vi "Handle Menu Selection.vi"(6 "Coords":T1, 8 "error in (no error)":errorcluster, 9 "Item Tag":string, 10 "Tree Refnum":refnum<vi>, 11 "Process Builder View in":refnum<class "Process Builder View.lvclass">) -> (0 "error out":errorcluster, 3 "Process Builder View out":refnum<class "Process Builder View.lvclass">)   [LabVIEW 2019, in "Process Builder View.lvclass"]
uses:
  <vilib>/gpm_packages/@cs/Car-wash/Source/Process Builder View/Process Builder View.lvclass
  C:/Program Files/National Instruments/LabVIEW 2019/vi.lib/gpm_packages/@cs/Test-executive-builder/Source/Test Executive Builder View/Test Executive Builder View/Test Executive Builder View.lvclass
  <vilib>/Utility/miscctls.llb/LVPoint32TypeDef.ctl
  <vilib>/gpm_packages/@cs/Test-executive-builder/Source/Test Executive Builder View/Test Executive Builder View/Test Executive Builder View.lvclass/Test Executive Builder View.ctl
  <vilib>/gpm_packages/@cs/Test-executive-builder/Source/Application Dependencies/Insert Test Step.ctl
  <vilib>/gpm_packages/@cs/Test-executive-builder/Source/Application Dependencies/Insert While Loop.ctl
  <vilib>/gpm_packages/@cs/Test-executive-builder/Source/Application Dependencies/Insert For Loop.ctl
  <vilib>/gpm_packages/@cs/Test-executive-builder/Source/Application Dependencies/Insert Stop Loop.ctl
  <vilib>/gpm_packages/@cs/Test-executive-builder/Source/Application Dependencies/Insert Subroutine.ctl
  <vilib>/gpm_packages/@cs/Test-executive-builder/Source/Application Dependencies/Insert Subsequence.ctl
  <vilib>/gpm_packages/@cs/Test-executive-builder/Source/Application Dependencies/Insert Conditional.ctl
  <vilib>/gpm_packages/@cs/Test-executive-builder/Source/Test Executive Builder View/Tree Click Interpreter/Tree Click Interpreter.lvclass
  <vilib>/gpm_packages/@cs/Test-executive-builder/Source/Test Executive Builder View/Test Executive Builder View/Test Executive Builder View.lvclass
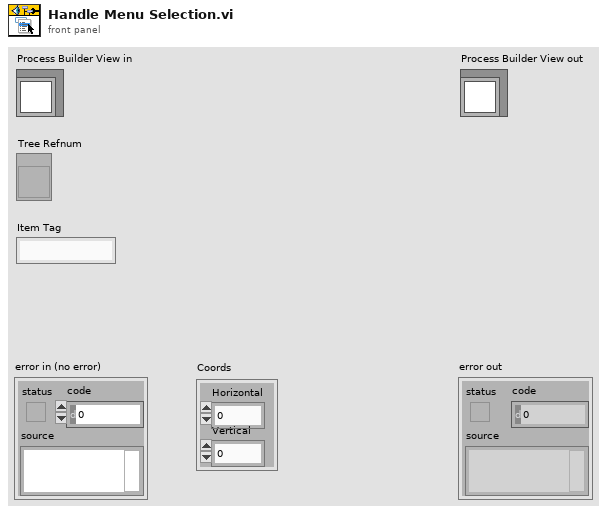
[diagram p1: front panel]
types:
  T1 = typedef "LVPoint32TypeDef.ctl" = cluster{"Horizontal":i32, "Vertical":i32}
  T2 = typedef "Insert Test Step.ctl" = cluster{"Parent ID":string, "Insertion Index":i32, "Test Step":string}
  T3 = typedef "Insert While Loop.ctl" = cluster{"Parent ID":string, "Insertion Index":i32}
  T4 = typedef "Insert For Loop.ctl" = cluster{"Parent ID":string, "Insertion Index":i32, "Iterations":i32}
  T5 = typedef "Insert Stop Loop.ctl" = cluster{"Parent ID":string, "Insertion Index":i32}
  T6 = typedef "Insert Subroutine.ctl" = cluster{"Parent ID":string, "Insertion Index":i32, "Path":path}
  T7 = typedef "Insert Subsequence.ctl" = cluster{"Parent ID":string, "Insertion Index":i32}
  T8 = typedef "Insert Conditional.ctl" = cluster{"Parent ID":string, "Insertion Index":i32}
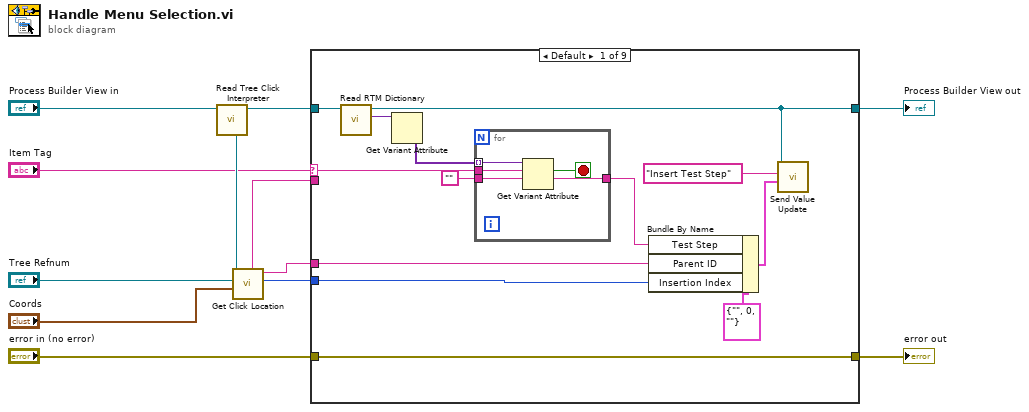
[diagram p0: block diagram]
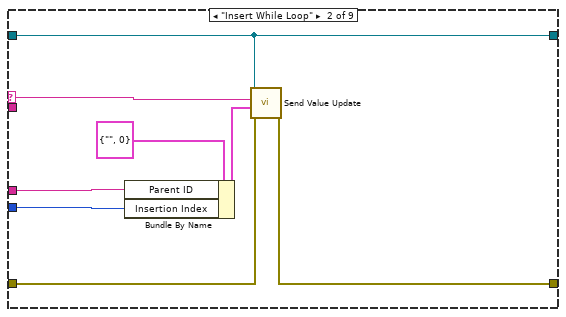
[diagram p2: hidden frame]
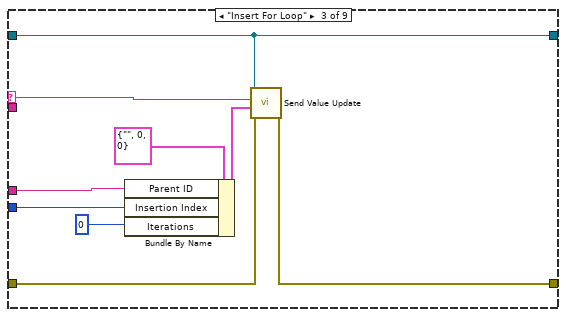
[diagram p3: hidden frame]
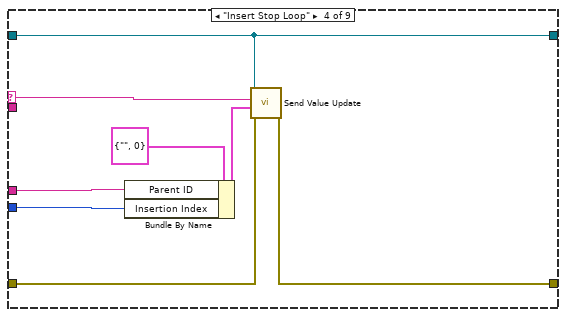
[diagram p4: hidden frame]
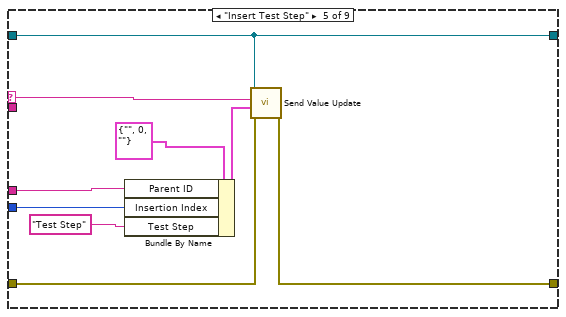
[diagram p5: hidden frame]
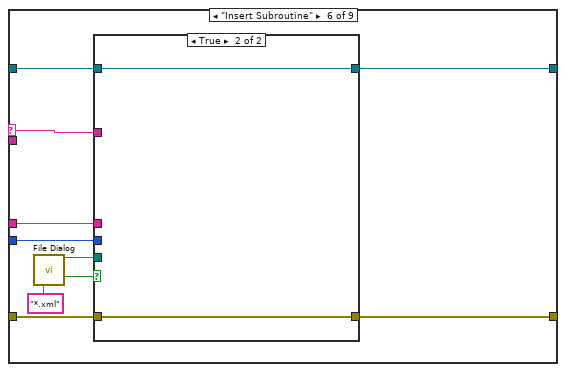
[diagram p6: hidden frame]
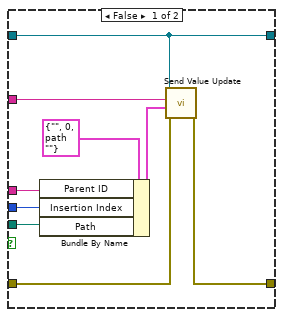
[diagram p7: hidden frame]
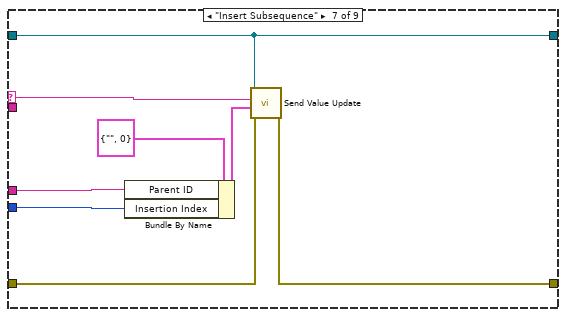
[diagram p8: hidden frame]
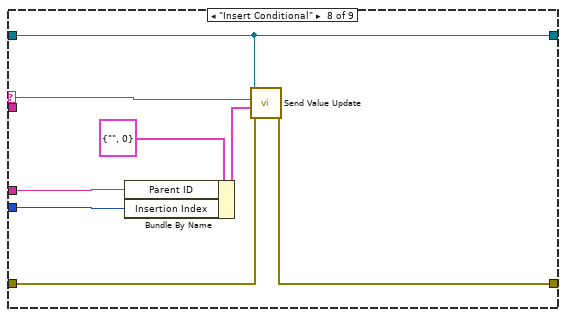
[diagram p9: hidden frame]
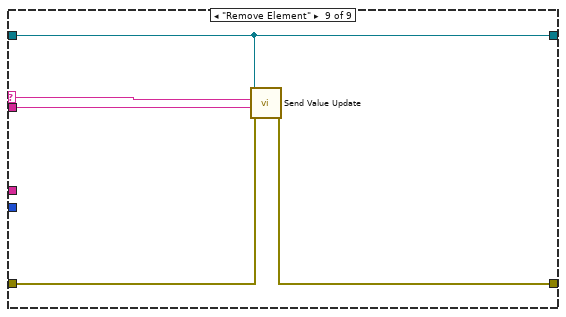
[diagram p10: hidden frame]
diagram:
  n1 = call <vilib>:"Read Tree Click Interpreter.vi"("Test Executive Builder View in"="Process Builder View in") -> ("Test Executive Builder View out"=w12:refnum<class "Process Builder View.lvclass">, "Tree Click Interpreter"=w11:refnum<class "Tree Click Interpreter.lvclass">)  [unwired: 9 in]
  n2 = call-dynamic "Get Click Location.vi"("Coords"="Coords", "Tree Refnum"="Tree Refnum", "Tree Click Interpreter in"=w11) -> ("Insertion Index"=w10:i32, "Parent ID"=w9:string, "Tag"=w8:string)  [unwired: 4 in, 2 out]
  n3 = case shown="Default" "Item Tag" {
    selector: "Item Tag" -> [w21 w35 w44 w52 w61 w71 w90 w98 w103]
    tunnel: [w19 w38 w47 w55 w64 w66 w93 w101 w106] -> w6
    tunnel: w12 -> [w24 w38 w47 w55 w64 w74 w93 w101 w106]
    tunnel: [w25 w36 w45 w53 w62 w72 w91 w99 w104] -> w4
    tunnel: "error in (no error)" -> [w25 w37 w46 w54 w63 w73 w92 w100 w105]
    tunnel: w10 -> [w13 w34 w43 w51 w60 w70 w89 w97 _]
    tunnel: w9 -> [w14 w33 w42 w50 w59 w69 w88 w96 _]
    tunnel: w8 -> [_ _ _ _ _ _ _ _ w102]
    frame Default {
      n4 = call <vilib>:"Read RTM Dictionary.vi"("Test Executive Builder View in"=w24) -> ("RTM Dictionary"=w23:variant, "Test Executive Builder View out"=w19:refnum<class "Process Builder View.lvclass">)  [unwired: 9 in]
      n5 = Get Variant Attribute(Variant=w23) -> (values=w22:variant[])  [unwired: 3 in, 3 out]
      n6 = for {
        tunnel: w22 -> [w30] mode=indexing
        tunnel: w21 -> [w29]
        tunnel: "" -> [w28]
        tunnel: [w26] -> w16
        stop <- w27 stop-if-true
        n7 = Get Variant Attribute(Variant=w30, name=w29, default value (empty Variant)=w28) -> (found=w27:bool, value=w26:string)  [unwired: 1 in, 2 out]
      }
      n8 = Bundle By Name(cluster=T2 {"Parent ID"="", "Insertion Index"=0, "Test Step"=""} ("Insert Test Step"), "Test Step"=w16, "Parent ID"=w14, "Insertion Index"=w13) -> (w15:T2)
      n9 = call-dynamic "Send Value Update.vi"("Value"=w15, "Datum Name"="Insert Test Step", "IViewable in"=w19) -> ()  [unwired: 8 in, 1 out]
    }
    frame "Insert While Loop" {
      n10 = Bundle By Name(cluster=T3 {"Parent ID"="", "Insertion Index"=0} ("Insert While Loop"), "Parent ID"=w33, "Insertion Index"=w34) -> (w31:T3)
      n11 = call-dynamic "Send Value Update.vi"("error in (no error)"=w37, "Value"=w31, "Datum Name"=w35, "IViewable in"=w38) -> ("error out"=w36:errorcluster)  [unwired: 7 in]
    }
    frame "Insert For Loop" {
      n12 = Bundle By Name(cluster=T4 {"Parent ID"="", "Insertion Index"=0, "Iterations"=0} ("Insert For Loop"), "Parent ID"=w42, "Insertion Index"=w43, "Iterations"=0) -> (w41:T4)
      n13 = call-dynamic "Send Value Update.vi"("error in (no error)"=w46, "Value"=w41, "Datum Name"=w44, "IViewable in"=w47) -> ("error out"=w45:errorcluster)  [unwired: 7 in]
    }
    frame "Insert Stop Loop" {
      n14 = Bundle By Name(cluster=T5 {"Parent ID"="", "Insertion Index"=0} ("Insert Stop Loop"), "Parent ID"=w50, "Insertion Index"=w51) -> (w49:T5)
      n15 = call-dynamic "Send Value Update.vi"("error in (no error)"=w54, "Value"=w49, "Datum Name"=w52, "IViewable in"=w55) -> ("error out"=w53:errorcluster)  [unwired: 7 in]
    }
    frame "Insert Test Step" {
      n16 = Bundle By Name(cluster=T2 {"Parent ID"="", "Insertion Index"=0, "Test Step"=""} ("Insert Test Step"), "Parent ID"=w59, "Insertion Index"=w60, "Test Step"="Test Step") -> (w58:T2)
      n17 = call-dynamic "Send Value Update.vi"("error in (no error)"=w63, "Value"=w58, "Datum Name"=w61, "IViewable in"=w64) -> ("error out"=w62:errorcluster)  [unwired: 7 in]
    }
    frame "Insert Subroutine" {
      n18 = call "File Dialog"("pattern (all files)"="*.xml") -> ("selected path"=w68:path, "cancelled"=w65:bool)  [unwired: 11 in, 2 out]
      n19 = case shown="True" w65 {
        tunnel: w74 -> [w75 w85]
        tunnel: w73 -> [w83 w84]
        tunnel: [w82 w84] -> w72
        tunnel: w71 -> [w81 _]
        tunnel: w70 -> [w80 _]
        tunnel: w69 -> [w79 _]
        tunnel: w68 -> [w76 _]
        tunnel: [w75 w85] -> w66
        frame False {
          n20 = Bundle By Name(cluster=T6 {"Parent ID"="", "Insertion Index"=0, "Path"=path ""} ("Insert Subroutine"), "Parent ID"=w79, "Insertion Index"=w80, "Path"=w76) -> (w78:T6)
          n21 = call-dynamic "Send Value Update.vi"("error in (no error)"=w83, "Value"=w78, "Datum Name"=w81, "IViewable in"=w75) -> ("error out"=w82:errorcluster)  [unwired: 7 in]
        }
        frame True {
        }
      }
    }
    frame "Insert Subsequence" {
      n22 = Bundle By Name(cluster=T7 {"Parent ID"="", "Insertion Index"=0} ("Insert Subsequence"), "Parent ID"=w88, "Insertion Index"=w89) -> (w87:T7)
      n23 = call-dynamic "Send Value Update.vi"("error in (no error)"=w92, "Value"=w87, "Datum Name"=w90, "IViewable in"=w93) -> ("error out"=w91:errorcluster)  [unwired: 7 in]
    }
    frame "Insert Conditional" {
      n24 = Bundle By Name(cluster=T8 {"Parent ID"="", "Insertion Index"=0} ("Insert Conditional"), "Parent ID"=w96, "Insertion Index"=w97) -> (w95:T8)
      n25 = call-dynamic "Send Value Update.vi"("error in (no error)"=w100, "Value"=w95, "Datum Name"=w98, "IViewable in"=w101) -> ("error out"=w99:errorcluster)  [unwired: 7 in]
    }
    frame "Remove Element" {
      n26 = call-dynamic "Send Value Update.vi"("error in (no error)"=w105, "Value"=w102, "Datum Name"=w103, "IViewable in"=w106) -> ("error out"=w104:errorcluster)  [unwired: 7 in]
    }
  }
  "error out" <- w4
  "Process Builder View out" <- w6
